vi "Post Build.vi"   [LabVIEW 2016]
uses:
  <userlib>/LevyLab/PostBuildSupport/PostBuildSupport.lvclass
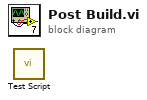
[diagram p0: block diagram]
diagram:
  n1 = call <userlib>:"Test Script.vi"() -> ()  [unwired: 12 in]
